vi "CloseDevice.vi"(10 "DevIndex":u32, 11 "DevType":u32) -> (5 "CloseDevice_Success?":u32)   [LabVIEW 2016]
uses:
  ECanVci.dll
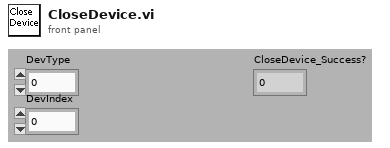
[diagram p1: front panel]
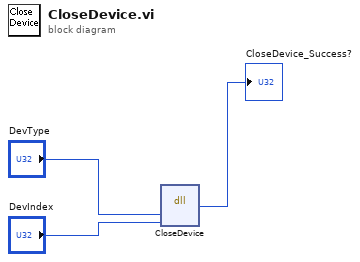
[diagram p0: block diagram]
diagram:
  n1 = dll-call lib="C:/Users/Azmat/Desktop/Labview/ECanVci.dll" fn="CloseDevice"("DevType"="DevType", "DevIndex"="DevIndex") -> ("CloseDevice_Success"=→"CloseDevice_Success?":u32)  [unwired: 5 in, 2 out]
